vi "Reactive Power Setpoint.vi"(8 "error in":errorcluster, 10 "DER_SetPointQ":T1, 11 "Manual Control in":refnum<class "Manual Control.lvclass">) -> (0 "error out":errorcluster, 3 "Manual Control out":refnum<class "Manual Control.lvclass">)   [LabVIEW 2018, in "Manual Control Actor.lvlib" / "Manual Control.lvclass"]
uses:
  Manual Control.lvclass
  C:/Users/Administrator/Desktop/2018LabVIEW EMS/Device Communication and Control Abstract Actor/Device Communication and Control Abstract/Device Communication and Control Abstract.lvclass
  <vilib>/ORNL/CSEISMIC DDS/CSEISMIC DDS Base/Data Types/DER_SetPointQ.ctl
  <vilib>/ORNL/CSEISMIC DDS/CSEISMIC DDS Base/Data Types/Controls/DeviceID.ctl
  Manual Control.lvclass/Manual Control.ctl
  <vilib>/ActorFramework/Actor/Actor.lvclass/Actor.ctl
  Device Communication and Control Abstract Actor/Device Communication and Control Abstract/Device Communication and Control Abstract.lvclass/Device Communication and Control Abstract.ctl
  Device Communication and Control Abstract Actor/Device Communication and Control Abstract Messages/Set DER SetPointQ Msg/Set DER SetPointQ Msg.lvclass/Set DER SetPointQ Msg.ctl
  <vilib>/ActorFramework/Message Enqueuer/Message Enqueuer.lvclass/Message Enqueuer.ctl
  Device Communication and Control Abstract Actor/Device Communication and Control Abstract Messages/Set DER SetPointQ Msg/Send Set DER SetPointQ.vi
  <vilib>/ActorFramework/Actor/Read Caller Enqueuer.vi
  <vilib>/ActorFramework/Message Enqueuer/Enqueue.vi
  Device Communication and Control Abstract Actor/Device Communication and Control Abstract/Device Communication and Control Abstract.lvclass
  C:/Program Files (x86)/National Instruments/LabVIEW 2018/vi.lib/ActorFramework/Actor/Actor.lvclass
  Device Communication and Control Abstract Actor/Device Communication and Control Abstract Messages/Set DER SetPointQ Msg/Set DER SetPointQ Msg.lvclass
  C:/Program Files (x86)/National Instruments/LabVIEW 2018/vi.lib/ActorFramework/Message/Message.lvclass
  <vilib>/ActorFramework/Message Priority Queue/Priority Enqueue.vi
  <vilib>/ORNL/CSEISMIC DDS/CSEISMIC DDS Base/CSEISMIC DDS.lvclass
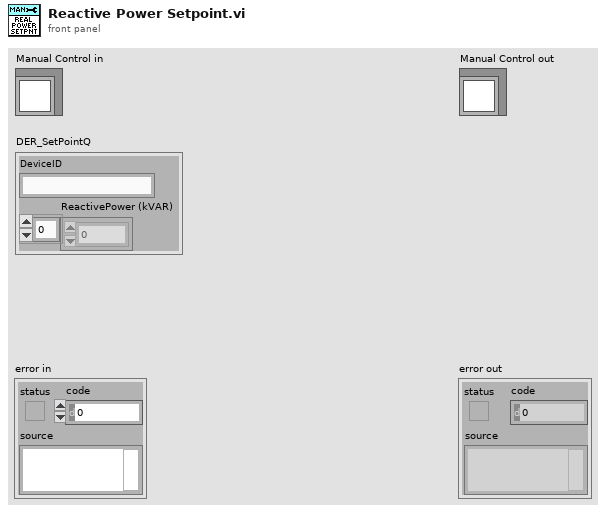
[diagram p1: front panel]
types:
  T1 = typedef "CSEISMIC DDS.lvlib/CSEISMIC DDS.lvclass/DER_SetPointQ.ctl" = cluster{"DeviceID":T2, "ReactivePower (kVAR)":dbl[]}
  T2 = typedef "CSEISMIC DDS.lvlib/CSEISMIC DDS.lvclass/DeviceID.ctl" = string
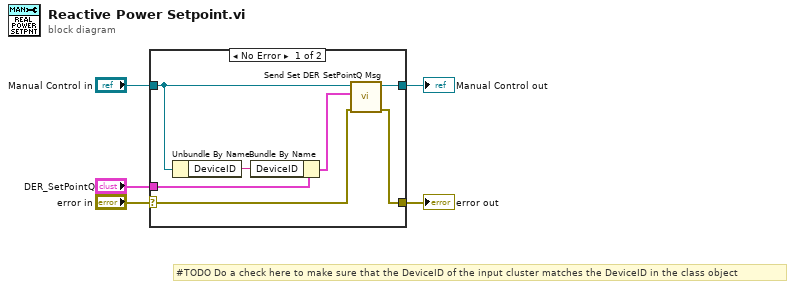
[diagram p0: block diagram]
diagram:
  # "#TODO Do a check here to make sure that the DeviceID of the input cluster matches the DeviceID in the class object"
  n1 = case shown="No Error" "error in" {
    selector: "error in" -> [w7 w14]
    tunnel: [w6 w14] -> w4
    tunnel: [w9 w13] -> w2
    tunnel: "Manual Control in" -> [w10 w13]
    tunnel: "DER_SetPointQ" -> [w12 _]
    frame No Error {
      n2 = Unbundle By Name(w10) -> ("DeviceID"=w11:T2)
      n3 = Bundle By Name(cluster=w12, "DeviceID"=w11) -> (w8:T1)
      n4 = call "Send Set DER SetPointQ Msg.vi"("error in"=w7, "DER_SetPointQ"=w8, "SCADA Sub Abstract in"=w10) -> ("error out"=w6:errorcluster, "dup SCADA Sub Abstract"=w9:refnum<class "Manual Control.lvclass">)  [unwired: 7 in]
    }
    frame Error {
    }
  }
  "error out" <- w4
  "Manual Control out" <- w2
